vi "Is Nework.vi"(10 "Set":set{string}(c389), 11 "NetAn in":refnum<class "NetAn.lvclass">) -> (2 "Is network":bool, 3 "NetAn out":refnum<class "NetAn.lvclass">)   [LabVIEW 2020, in "NetAn.lvclass"]
uses:
  NetAn.lvclass
  NetAn.lvclass/NetAn.ctl
  Global 1.vi
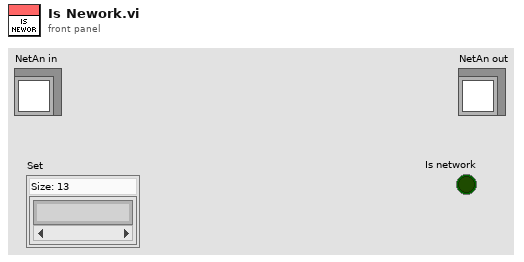
[diagram p1: front panel]
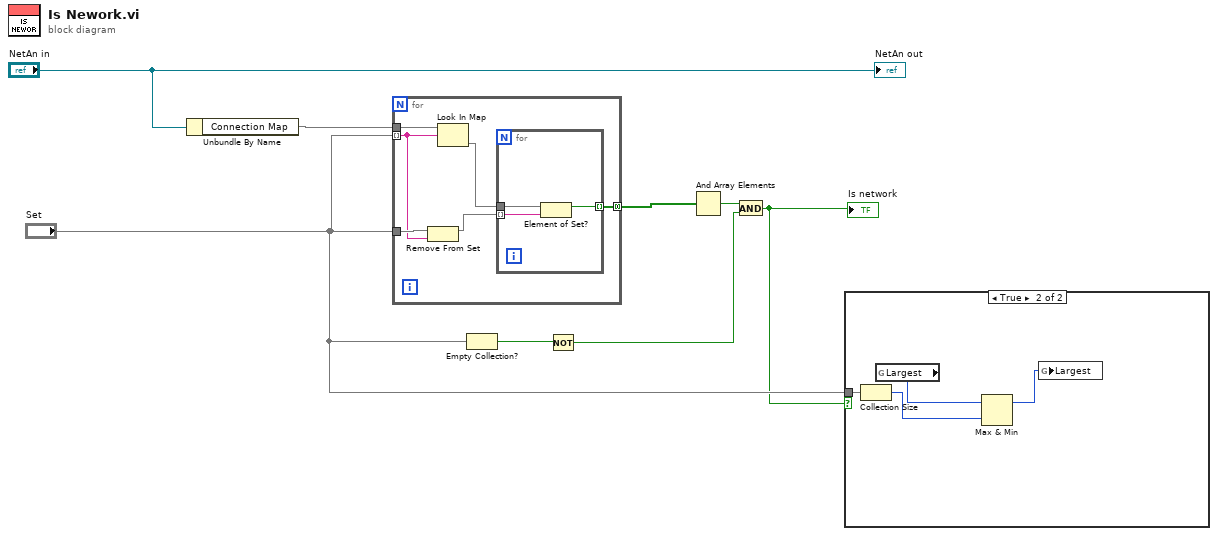
[diagram p0: block diagram]
diagram:
  n1 = Unbundle By Name("NetAn in") -> ("Connection Map"=w7:map{string, set{string}})
  n2 = for {
    tunnel: w7 -> [w14]
    tunnel: "Set" -> [w11] mode=indexing
    tunnel: "Set" -> [w12]
    tunnel: [w9] -> w6 mode=concatenating
    n3 = Remove From Set(10:w11, 11:w12) -> (3:w10:set{string})  [unwired: 1 out]
    n4 = Look In Map(map=w14, key=w11) -> (value=w13:set{string})  [unwired: 1 in, 1 out]
    n5 = for {
      tunnel: w13 -> [w17]
      tunnel: w10 -> [w16] mode=indexing
      tunnel: [w15] -> w9 mode=indexing
      n6 = Element of Set?(10:w16, 11:w17) -> (3:w15:bool)
    }
  }
  n7 = Empty Collection?(1:"Set") -> (0:w4:bool)
  n8 = Not(x=w4) -> (.not. x?=w3:bool)
  n9 = And Array Elements(Boolean array=w6) -> (logical AND=w5:bool)
  n10 = And(x=w5, y=w3) -> (x .and. y?=w1:bool)
  "Is network" <- w1
  n11 = case shown="True" w1 {
    tunnel: "Set" -> [_ w21]
    frame False {
    }
    frame True {
      n12 = Collection Size(1:w21) -> (0:w19:i32)
      n13 = global read "Global 1.vi" "Largest"() -> (w20:i32)
      n14 = Max & Min(x=w20, y=w19) -> (max(x,y)=w18:i32)  [unwired: 1 out]
      n15 = global write "Global 1.vi" "Largest"(w18) -> ()
    }
  }
  "NetAn out" <- "NetAn in"
